vi "OpenTransit.vi"(7 "Inhibit":bool, 9 "WhatAroundMe? Clean":cluster{"T":dbl, "Range":dbl, "Bearing":dbl}[](array[cluster]), 11 "Velocity":dbl) -> (2 "ActCommand":dbl[](array[numeric]), 4 "InhibitOut":bool, 10 "Boat":T1)   [LabVIEW 2011]
doc: "This subVI executes a wall folowing Midbrain behaviors. Its inputs are the outputs of the three SENSE processes, the overall velocity requested of the robot, a suppression value from another co-brahvior and an inhibit signal to turn the behavior off. The outputs are a 90 element steering array, a suppression value to diminish the output of co-behaviors and an inhibit output to shut off otehr behaviors.\n\nIt is designed to work with a 90 element behavior arbiter."
uses:
  WhereAmI.ctl
panel:
  # "This VI contains a wall following behavior at the Midbrain level"
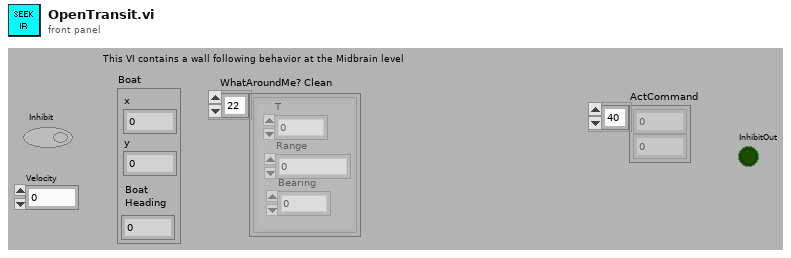
[diagram p1: front panel]
types:
  T1 = typedef "WhereAmI.ctl" = cluster{"x":sgl, "y":sgl, "Boat\nHeading":sgl}
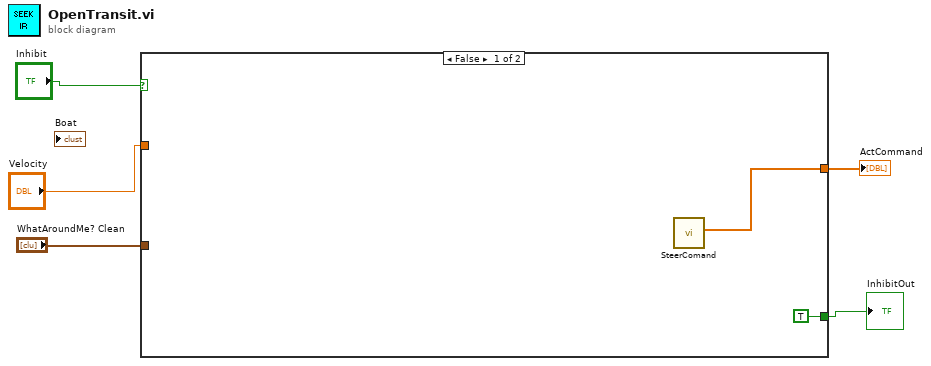
[diagram p0: block diagram]
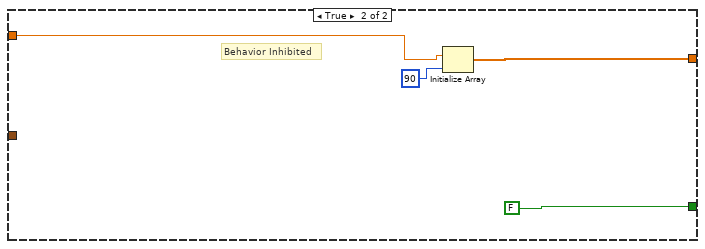
[diagram p2: hidden frame]
diagram:
  n1 = case shown="False" "Inhibit" {
    tunnel: "Velocity" -> [_ w8]
    tunnel: "WhatAroundMe? Clean" -> [_ _]
    tunnel: [w6 w10] -> w2
    tunnel: [TRUE ("InhibitOut") FALSE ("InhibitOut")] -> w1
    frame False {
      n2 = call "SteerComand.vi"() -> ("ManualActCommand"=w6:dbl[])  [unwired: 11 in]
    }
    frame True {
      # "Behavior Inhibited"
      n3 = Initialize Array "Initialize Array"(w8, 90 ("dimension size")) -> (w10:dbl[])
    }
  }
  "ActCommand" <- w2
  "InhibitOut" <- w1
